vi "Read Connected.vi"(8 "error in (no error)":errorcluster, 11 "ClientBase in":refnum<class "TCP.lvclass">) -> (0 "error out":errorcluster, 2 "Connected":bool, 3 "ClientBase out":refnum<class "TCP.lvclass">)   [LabVIEW 2020, in "TCP.lvlib" / "TCP.lvclass"]
uses:
  TCP.lvclass
  TCP.lvclass/TCP.ctl
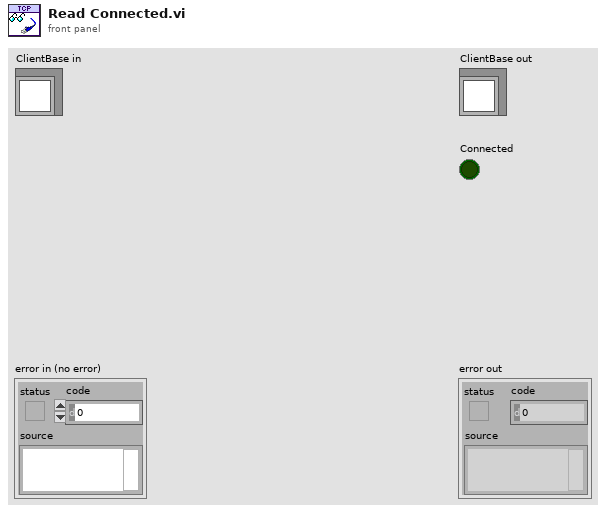
[diagram p1: front panel]
types:
  T1 = typedef "ConnectionProperties.ctl" = cluster{"Address":string, "Port":u16, "ID":string, "Connection ID":refnum<k5>, "Connected":bool, "Abort":bool}
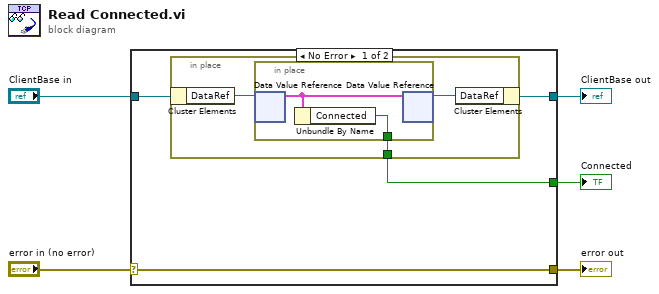
[diagram p0: block diagram]
diagram:
  n1 = case shown="No Error" "error in (no error)" {
    selector: "error in (no error)" -> [w9 w15]
    tunnel: [w9 w15] -> w4
    tunnel: [w7 w16] -> w2
    tunnel: "ClientBase in" -> [w8 w16]
    tunnel: [w6 _] -> w1
    frame No Error {
      n2 = in-place {
        in-place-border: [w10] -> w6
        n3 = in-place-cluster #1(w8) -> ("DataRef"=w12:refnum<data-value>)
        n4 = in-place {
          in-place-border: [w13] -> w10
          n5 = in-place-dvr #2(w12) -> (w14:T1)  [unwired: 1 out]
          n6 = Unbundle By Name(w14) -> ("Connected"=w13:bool)
          n7 = in-place-dvr #2(w14) -> (w11:refnum<data-value>)  [unwired: 1 out]
        }
        n8 = in-place-cluster #1("DataRef"=w11) -> (w7:refnum<class "TCP.lvclass">)
      }
    }
    frame Error {
    }
  }
  "error out" <- w4
  "ClientBase out" <- w2
  "Connected" <- w1
